vi "Instr_InitObject.vi"(8 "error in (no error)":errorcluster, 9 "Instrument Configuration":variant, 10 "Instrument address":refnum<visa-resource-name>, 11 "HP34401A in":refnum<class "HP34401A.lvclass">) -> (0 "error out":errorcluster, 3 "HP34401A out":refnum<class "HP34401A.lvclass">)   [LabVIEW 2019, in "HP34401A.lvclass"]
uses:
  HP34401A.lvclass
  HP34401A_CommandsGlobal.vi
  MultimeterControl.lvclass
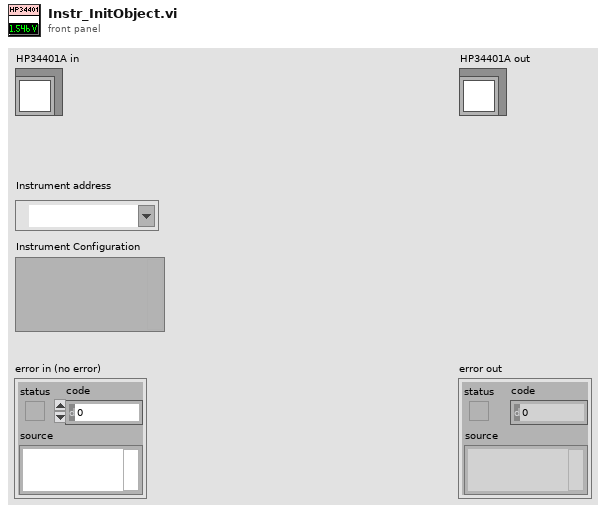
[diagram p1: front panel]
types:
  T1 = cluster{"Instrument name":string, "Command \"Reset\"":string, "Command \"Initialise\"":string, "Command \"Read Data\"":string}
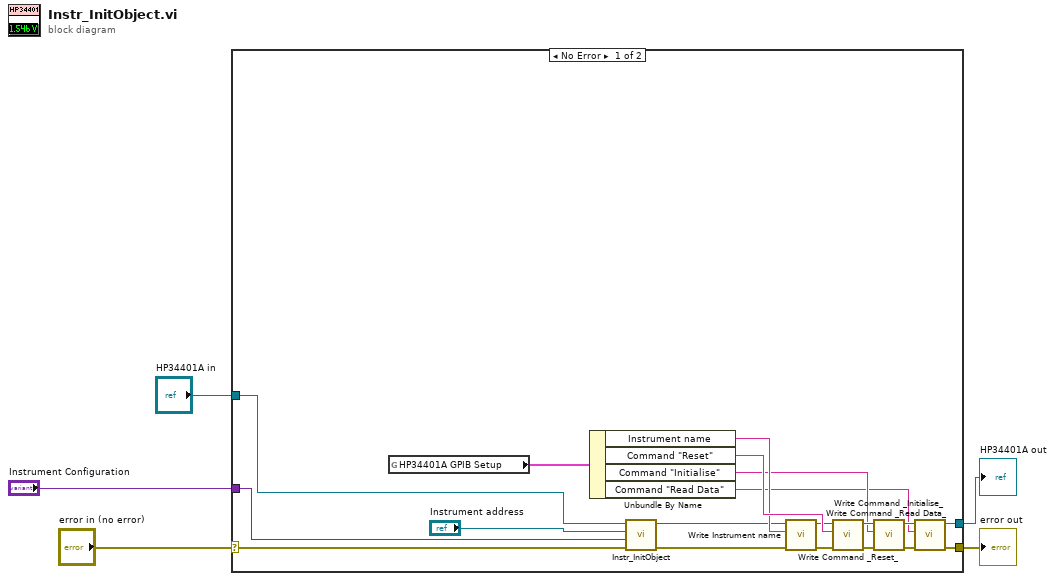
[diagram p0: block diagram]
diagram:
  n1 = case shown="No Error" "error in (no error)" {
    selector: "error in (no error)" -> [w13 w26]
    tunnel: [w21 w26] -> w5
    tunnel: "HP34401A in" -> [w15 w25]
    tunnel: [w18 w25] -> w3
    tunnel: "Instrument Configuration" -> [w9 _]
    frame No Error {
      n2 = global read "HP34401A_CommandsGlobal.vi" "HP34401A GPIB Setup"() -> (w8:T1)
      n3 = Unbundle By Name(w8) -> ("Instrument name"=w17:string, "Command \"Reset\""=w24:string, "Command \"Initialise\""=w7:string, "Command \"Read Data\""=w6:string)
      n4 = call-parent "Instr_InitObject.vi"("error in (no error)"=w13, "Instrument Configuration"=w9, "Instrument address"="Instrument address", "MultimeterControl in"=w15) -> ("error out"=w12:errorcluster, "MultimeterControl out"=w14:refnum<class "HP34401A.lvclass">)  [unwired: 6 in]
      n5 = call-dynamic "Write Instrument name.vi"("error in (no error)"=w12, "Instrument name"=w17, "InstControl in"=w14) -> ("error out"=w10:errorcluster, "InstControl out"=w11:refnum<class "HP34401A.lvclass">)  [unwired: 7 in]
      n6 = call-dynamic "Write Command _Reset_.vi"("error in (no error)"=w10, "Command \"Reset\""=w24, "MultimeterControl in"=w11) -> ("error out"=w23:errorcluster, "MultimeterControl out"=w20:refnum<class "HP34401A.lvclass">)  [unwired: 7 in]
      n7 = call-dynamic "Write Command _Initialise_.vi"("error in (no error)"=w23, "Command \"Initialise\""=w7, "MultimeterControl in"=w20) -> ("error out"=w22:errorcluster, "MultimeterControl out"=w19:refnum<class "HP34401A.lvclass">)  [unwired: 7 in]
      n8 = call-dynamic "Write Command _Read Data_.vi"("error in (no error)"=w22, "Command \"Read Data\""=w6, "MultimeterControl in"=w19) -> ("error out"=w21:errorcluster, "MultimeterControl out"=w18:refnum<class "HP34401A.lvclass">)  [unwired: 7 in]
    }
    frame Error {
    }
  }
  "error out" <- w5
  "HP34401A out" <- w3
